vi "Configure And Set A Digital Port.vi"() -> ()   [LabVIEW 2020]
uses:
  <instrlib>/BDAQ-6104/Public/Data/Write Single Digital Port.vi
  <instrlib>/BDAQ-6104/BDAQ-6104.lvlib
panel:
  in  "Pin State":bool=TRUE
  in  "Pin Number":T1(ring)=enum."Digital Pin 3"
  in  "Pin Direction":T2(array[cluster])=[{"Pin Number"=enum."Digital Pin 0", "Pin State"=FALSE}, {"Pin Number"=enum."Digital Pin 1", "Pin State"=FALSE}, {"Pin Number"=enum."Digital Pin 2", "Pin State"=FALSE}, {"Pin Number"=enum."Digital Pin 3", "Pin State"=TRUE}]
  in  "VISA resource name":refnum<visa-resource-name>
  # "Configure Digital Pin 3 as an output and set the\nstate high (On, +5V)."
  # "Input"
  # "Output"
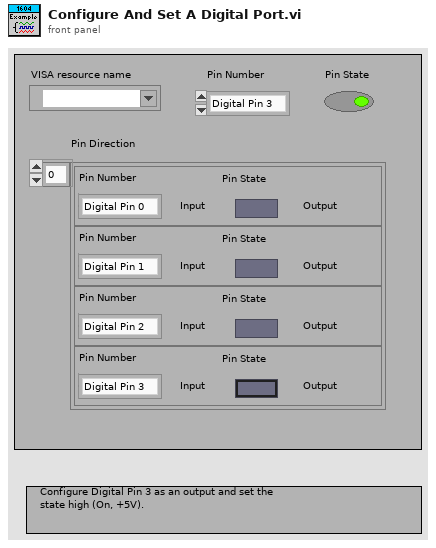
[diagram p1: front panel]
types:
  T1 = enum16{"Digital Pin 0", "Digital Pin 1", "Digital Pin 2", "Digital Pin 3"}
  T2 = cluster{"Pin Number":enum16{"Digital Pin 0", "Digital Pin 1", "Digital Pin 2", "Digital Pin 3"}, "Pin State":bool}[]
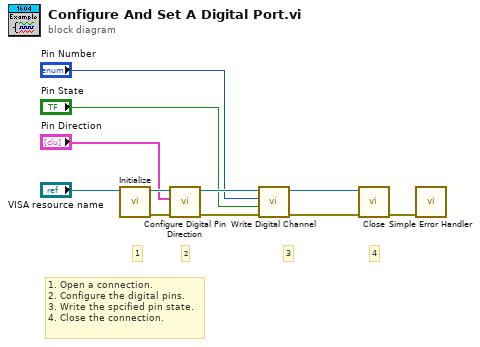
[diagram p0: block diagram]
diagram:
  # "1. Open a connection.\n2. Configure the digital pins.\n3. Write the spcified pin state.\n4. Close the connection."
  # "4"
  # "3"
  # "2"
  # "1"
  n1 = call <instrlib>:"Initialize.vi"("VISA resource name"="VISA resource name") -> ("error out"=w10:errorcluster, "VISA resource name out"=w11:refnum<visa-resource-name>)  [unwired: 9 in]
  n2 = call <instrlib>:"Configure Digital Pin Direction.vi"("error in (no error)"=w10, "Pin Direction"="Pin Direction", "VISA resource name"=w11) -> ("error in (no error) 2"=w6:errorcluster, "VISA resource name 2"=w7:refnum<visa-resource-name>)  [unwired: 7 in]
  n3 = call-poly <instrlib>:"Write Digital Channel.vi"("error in (no error)"=w6, "Pin State"="Pin State", "Pin Number"="Pin Number", "VISA resource name"=w7) -> ("error out"=w2:errorcluster, "VISA resource name out"=w3:refnum<visa-resource-name>)  [unwired: 6 in]
  n4 = call <instrlib>:"Close.vi"("error in (no error)"=w2, "VISA resource name"=w3) -> ("error out"=w1:errorcluster)  [unwired: 9 in]
  n5 = call <vilib>:"Simple Error Handler.vi"("error in (no error)"=w1) -> ()  [unwired: 4 in, 5 out]
